vi "mute.vi"(8 "error in (no error)":errorcluster, 11 "AdvancedRemote in":refnum<class "AdvancedRemote.lvclass">) -> (0 "error out":errorcluster, 3 "AdvancedRemote out":refnum<class "AdvancedRemote.lvclass">)   [LabVIEW 2017, in "AdvancedRemote.lvclass"]
uses:
  AdvancedRemote.lvclass
  ConsoleOut/Print Options.ctl
  Device Class/Device.lvclass
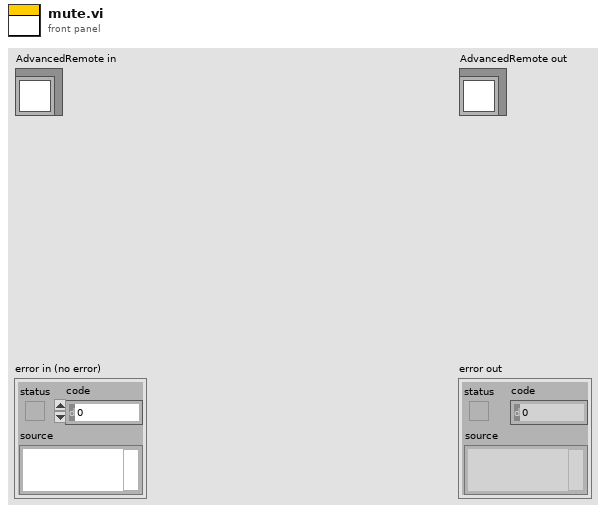
[diagram p1: front panel]
types:
  T1 = typedef "Print Options.ctl" = enum16{"Create", "Get Reference", "Print", "Print Header", "Close"}
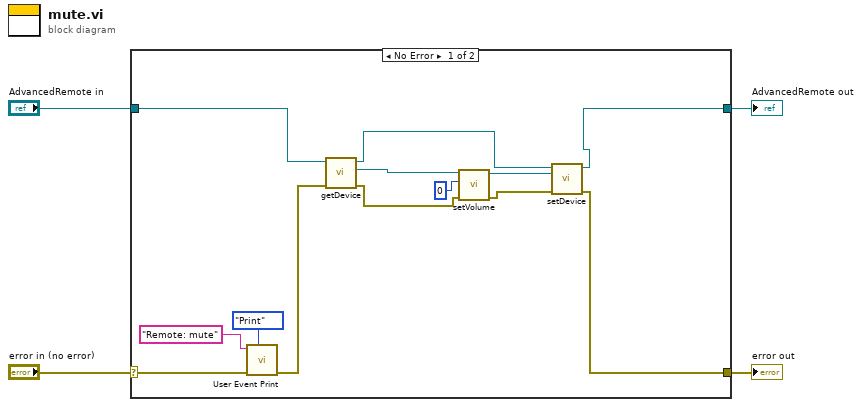
[diagram p0: block diagram]
diagram:
  n1 = case shown="No Error" "error in (no error)" {
    selector: "error in (no error)" -> [w17 w19]
    tunnel: [w6 w19] -> w3
    tunnel: [w11 w18] -> w1
    tunnel: "AdvancedRemote in" -> [w14 w18]
    frame No Error {
      n2 = call "User Event Print.vi"("Options"=Print_Options."Print", "error in (no error)"=w17, "String to Print"="Remote: mute" ("message")) -> ("error out"=w7:errorcluster)  [unwired: 7 in, 1 out]
      n3 = call-dynamic "getDevice.vi"("error in (no error)"=w7, "AdvancedRemote in"=w14) -> ("error out"=w9:errorcluster, "Device.lvclass"=w16:refnum<class "Device.lvclass">, "AdvancedRemote out"=w12:refnum<class "AdvancedRemote.lvclass">)  [unwired: 7 in]
      n4 = call-dynamic "setVolume.vi"("error in (no error)"=w9, "volume"=0, "Device in"=w16) -> ("error out"=w8:errorcluster, "Device out"=w13:refnum<class "Device.lvclass">)  [unwired: 7 in]
      n5 = call-dynamic "setDevice.vi"("error in (no error)"=w8, "Device.lvclass"=w13, "AdvancedRemote in"=w12) -> ("error out"=w6:errorcluster, "AdvancedRemote out"=w11:refnum<class "AdvancedRemote.lvclass">)  [unwired: 7 in]
    }
    frame Error {
    }
  }
  "error out" <- w3
  "AdvancedRemote out" <- w1
